vi "Generator get i set.vi"() -> ()   [LabVIEW 2014]
panel:
  out "Array 3":string[](array[string])
  out "size(s)":i32
  out "Array 2":variant[](array[variant])
  out "VI Name":string
  out "Array":string[](array[string])
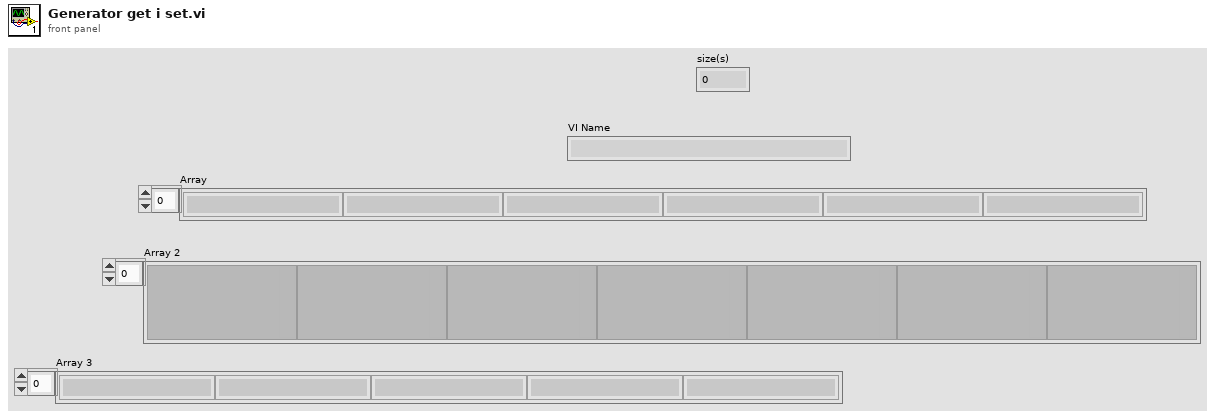
[diagram p1: front panel]
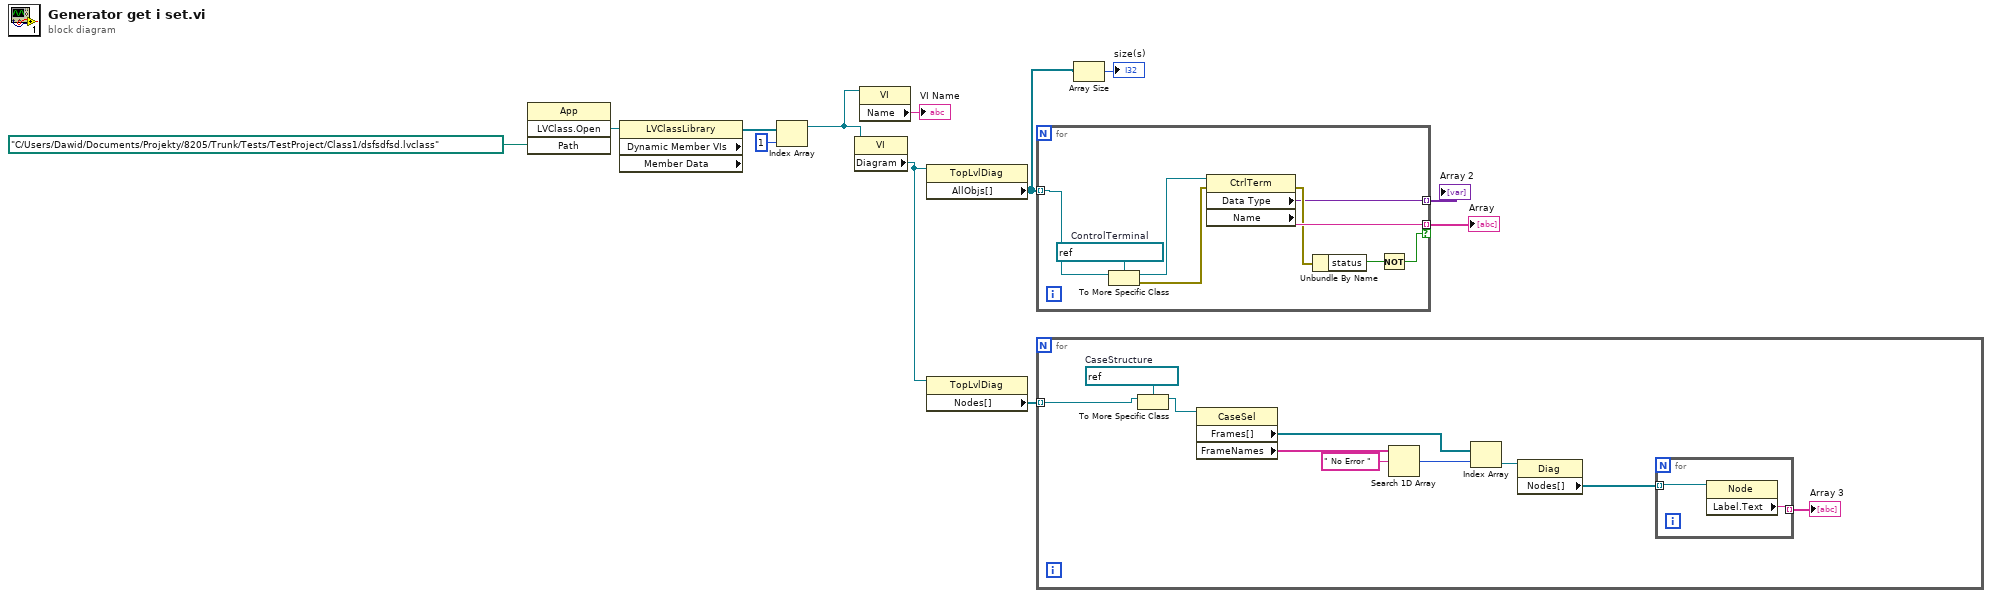
[diagram p0: block diagram]
diagram:
  n1 = invoke class="App" method="LVClass.Open"("Path"=path "C:/Users/Dawid/Documents/Projekty/8205/Trunk/Tests/TestProject/Class1/dsfsdfsd.lvclass" ("vi path")) -> ("LVClass.Open"=w11:refnum<vi>)  [unwired: 3 in, 3 out]
  n2 = property class="LVClassLibrary" props=["Dynamic Member VIs", "Member Data"](reference=w11) -> ("Dynamic Member VIs"=w10:refnum<vi>[])  [unwired: 1 in, 3 out]
  n3 = Index Array(array=w10, index=1) -> (element=w9:refnum<vi>)
  n4 = property class="VI"(reference=w9) -> ("Diagram"=w3:refnum<vi>)  [unwired: 1 in, 2 out]
  n5 = property class="VI"(reference=w9) -> ("Name"=→"VI Name":string)  [unwired: 1 in, 2 out]
  n6 = property class="TopLvlDiag"(reference=w3) -> ("AllObjs[]"=w2:refnum<vi>[])  [unwired: 1 in, 2 out]
  n7 = property class="TopLvlDiag"(reference=w3) -> ("Nodes[]"=w4:refnum<vi>[])  [unwired: 1 in, 2 out]
  n8 = for {
    tunnel: w2 -> [w18] mode=indexing
    tunnel: [w21] -> w7 mode=indexing if=w16
    tunnel: [w13] -> w5 mode=indexing
    w20 = refnum<vi> refnum  # ControlTerminal
    n9 = To More Specific Class(target class=w20, reference=w18) -> (specific class reference=w19:refnum<vi>, error out=w15:errorcluster)  [unwired: 1 in]
    n10 = property class="CtrlTerm"(reference=w19, error in=w15) -> (error out=w14:errorcluster, "Data Type"=w13:variant, "Name"=w21:string)  [unwired: 1 out]
    n11 = Unbundle By Name(w14) -> ("status"=w17:bool)
    n12 = Not(x=w17) -> (.not. x?=w16:bool)
  }
  "Array" <- w7
  "Array 2" <- w5
  n13 = for {
    tunnel: w4 -> [w30] mode=indexing
    w31 = refnum<vi> refnum  # CaseStructure
    n14 = To More Specific Class(target class=w31, reference=w30) -> (specific class reference=w29:refnum<vi>)  [unwired: 1 in, 1 out]
    n15 = property class="CaseSel"(reference=w29) -> ("Frames[]"=w25:refnum<vi>[], "FrameNames"=w28:string[])  [unwired: 1 in, 2 out]
    n16 = Search 1D Array(1D array=w28, element=" No Error ") -> (index of element=w26:i32)  [unwired: 1 in]
    n17 = Index Array(array=w25, index=w26) -> (element=w23:refnum<vi>)
    n18 = property class="Diag"(reference=w23) -> ("Nodes[]"=w24:refnum<vi>[])  [unwired: 1 in, 2 out]
    n19 = for {
      tunnel: w24 -> [w33] mode=indexing
      tunnel: [w32] -> w22 mode=indexing
      n20 = property class="Node"(reference=w33) -> ("Label.Text"=w32:string)  [unwired: 1 in, 2 out]
    }
    "Array 3" <- w22
  }
  n21 = Array Size(array=w2) -> (size(s)=→"size(s)":i32)
